vi "Write DLL path general.vi"   [LabVIEW 2016]
uses:
  DelayLine.lvclass
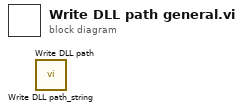
[diagram p0: block diagram]
diagram:
  n1 = call "Write DLL path_string.vi"() -> ()  [unwired: 10 in, 2 out]
  n2 = call "Write DLL path.vi"() -> ()  [unwired: 10 in, 2 out]
